vi "issue_ascii_command.vi"(0 "device_index (in) [0=def]":i32, 5 "Error In":errorcluster) -> (19 "Error Out":errorcluster)   [LabVIEW 2013, in "examples.lvlib"]
doc: "Demonstrates the usage of \"Send / Receive Command\" to issue ASCII commands to the referenced controller. This example demonstrates the key features required for any form of ASCII communications supported by the referenced controller.\n\nProduced By:\n\n<B>Kod Integrations, LLC</B>\n4835 Marianne Drive\nMount Airy, MD 21771\nhttp://www.kodintegrations.com\nemail: info@kodintegrations.com\nphone: (240) 687-1288"
uses:
  libraries/examples.lvlib
  classes/Controller/_Controller.lvclass
panel:
  out "success?":bool
  out "response (out)":string
  in  "ASCII Command (in)":string
  in  "clear_buffer? (T)":bool=TRUE
  # "instructions:\n\nSimply type in the ASCII command (as outlined in the\ndevice's ASCII Language Specification section of the \nmanual) and run the VI"
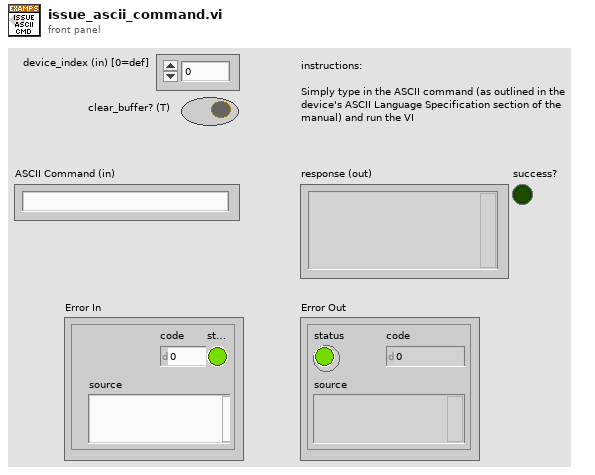
[diagram p1: front panel]
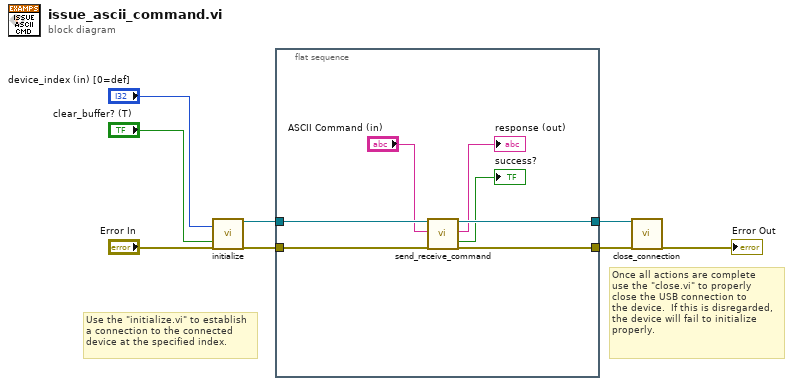
[diagram p0: block diagram]
diagram:
  # "Once all actions are complete\nuse the \"close.vi\" to properly\nclose the USB connection to \nthe device.  If this is disregarded,\nthe device will fail to initialize \nproperly."
  # "Use the \"initialize.vi\" to establish\na connection to the connected\ndevice at the specified index."
  n1 = call "initialize.vi"("device_index (in) [0=def]"="device_index (in) [0=def]", "clear_buffer? (T)"="clear_buffer? (T)", "error in (no error)"="Error In") -> ("reference (out)"=w5:refnum<class "_Controller.lvclass">, "error out"=w4:errorcluster)  [unwired: 15 in]
  n2 = flat-sequence {
    tunnel: w5 -> [w15]
    tunnel: w4 -> [w14]
    tunnel: [w12] -> w3
    tunnel: [w13] -> w2
    frame #0 {
      n3 = call "send_receive_command.vi"("reference (in)"=w15, "ASCII Command (in)"="ASCII Command (in)", "error in (no error)"=w14) -> ("reference (out)"=w12:refnum<class "_Controller.lvclass">, "response (out)"=→"response (out)":string, "success?"=→"success?":bool, "error out"=w13:errorcluster)  [unwired: 12 in, 1 out]
    }
  }
  n4 = call "close_connection.vi"("reference (in)"=w3, "error in (no error)"=w2) -> ("error out"=→"Error Out":errorcluster)  [unwired: 16 in, 1 out]
